vi "Draw.vi"(8 "Error In":errorcluster, 10 "PictureIn":picture, 11 "object in":refnum<class "HappyDecorator.lvclass">) -> (0 "Error Out":errorcluster, 2 "PictureOut":picture, 3 "object out":refnum<class "HappyDecorator.lvclass">)   [LabVIEW 2020, in "HappyDecorator.lvclass"]
uses:
  HappyDecorator.lvclass
  C:/Projects/DesignPatterns/DecoratorPattern2/ObjectDecorator_class/ObjectDecorator.lvclass
  Object_interface/Object.lvclass
  HappyDecorator.lvclass/HappyDecorator.ctl
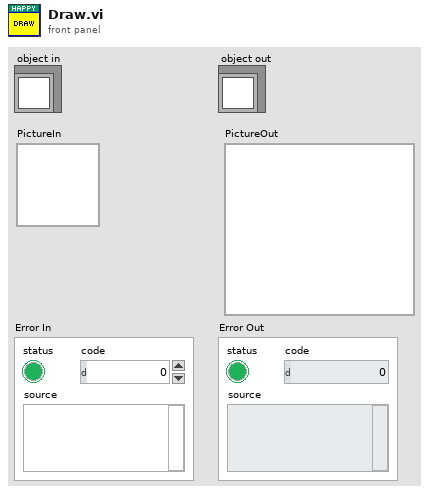
[diagram p1: front panel]
types:
  T1 = cluster{"Width":u16, "Style":enum32{"Solid", "Dash", "Dot", "DashDot", "DashDotDot"}}
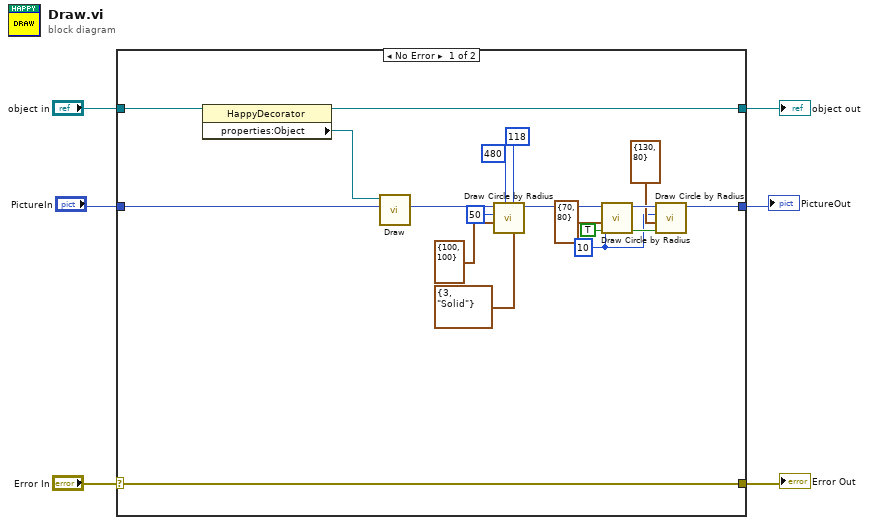
[diagram p0: block diagram]
diagram:
  n1 = case shown="No Error" "Error In" {
    selector: "Error In" -> [w24 w26]
    tunnel: [w24 w26] -> w5
    tunnel: [w22 w25] -> w3
    tunnel: "object in" -> [w23 w25]
    tunnel: "PictureIn" -> [w20 _]
    tunnel: [w11 _] -> w1
    frame No Error {
      w7 = i16 10 ("radius")
      w8 = TRUE ("fill?(F)")
      n2 = property class="HappyDecorator"(reference=w23) -> (reference out=w22:refnum<class "HappyDecorator.lvclass">, "properties:Object"=w21:refnum<class "Object.lvclass">)  [unwired: 1 in, 1 out]
      n3 = call-dynamic "Draw.vi"("PictureIn"=w20, "reference in"=w21) -> ("PictureOut"=w19:picture)  [unwired: 7 in, 2 out]
      n4 = call <vilib>:"Draw Circle by Radius.vi"("pen"=T1 {"Width"=3, "Style"=enum."Solid"}, "arc size(360)"=i16 118 ("start angle(0) 2"), "start angle(0)"=i16 480, "pixel center"=cluster{"horizontal":i16, "vertical":i16} {"horizontal"=100, "vertical"=100}, "radius"=i16 50, "picture"=w19) -> ("new picture"=w13:picture)  [unwired: 5 in]
      n5 = call <vilib>:"Draw Circle by Radius.vi"("fill?(F)"=w8, "pixel center"=cluster{"horizontal":i16, "vertical":i16} {"horizontal"=70, "vertical"=80}, "radius"=w7, "picture"=w13) -> ("new picture"=w12:picture)  [unwired: 7 in]
      n6 = call <vilib>:"Draw Circle by Radius.vi"("fill?(F)"=w8, "pixel center"=cluster{"horizontal":i16, "vertical":i16} {"horizontal"=130, "vertical"=80}, "radius"=w7, "picture"=w12) -> ("new picture"=w11:picture)  [unwired: 7 in]
    }
    frame Error {
    }
  }
  "Error Out" <- w5
  "object out" <- w3
  "PictureOut" <- w1
